vi "Auto Resize All Tree Columns (Uniform Text).vi"(6 "IngoreCols(Empty as default)":i32[](array[numeric]), 8 "error in (no error)":errorcluster, 11 "Tree Control":refnum<vi>) -> (0 "error out":errorcluster, 3 "Tree Control":refnum<vi>)   [LabVIEW 2017, in "csm-ui-support.lvlib"]
doc: "This VI resizes each column of the Tree specified by Tree Ref based on the widest entry of the column. Additionally, the array based on the Tree can be calculated according to the Tree Ref, which don't need additional input."
uses:
  csm-ui-support.lvlib
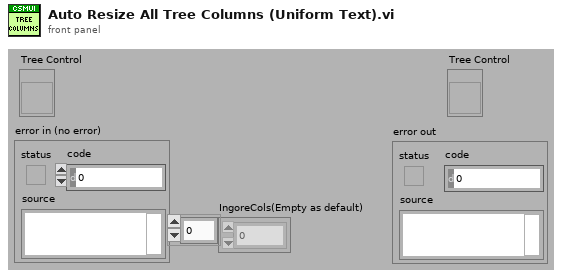
[diagram p1: front panel]
types:
  T1 = cluster{"Font Name:":string, "Size":i16, "Strikeout?":bool, "Italic?":bool, "Underline?":bool, "Outline?":bool, "Shadow?":bool, "Bold?":bool}
  T2 = enum16{"User-specified Font", "Application Font", "System Font", "Dialog Font"}
  T3 = cluster{"left":i16, "top":i16, "right":i16, "bottom":i16}
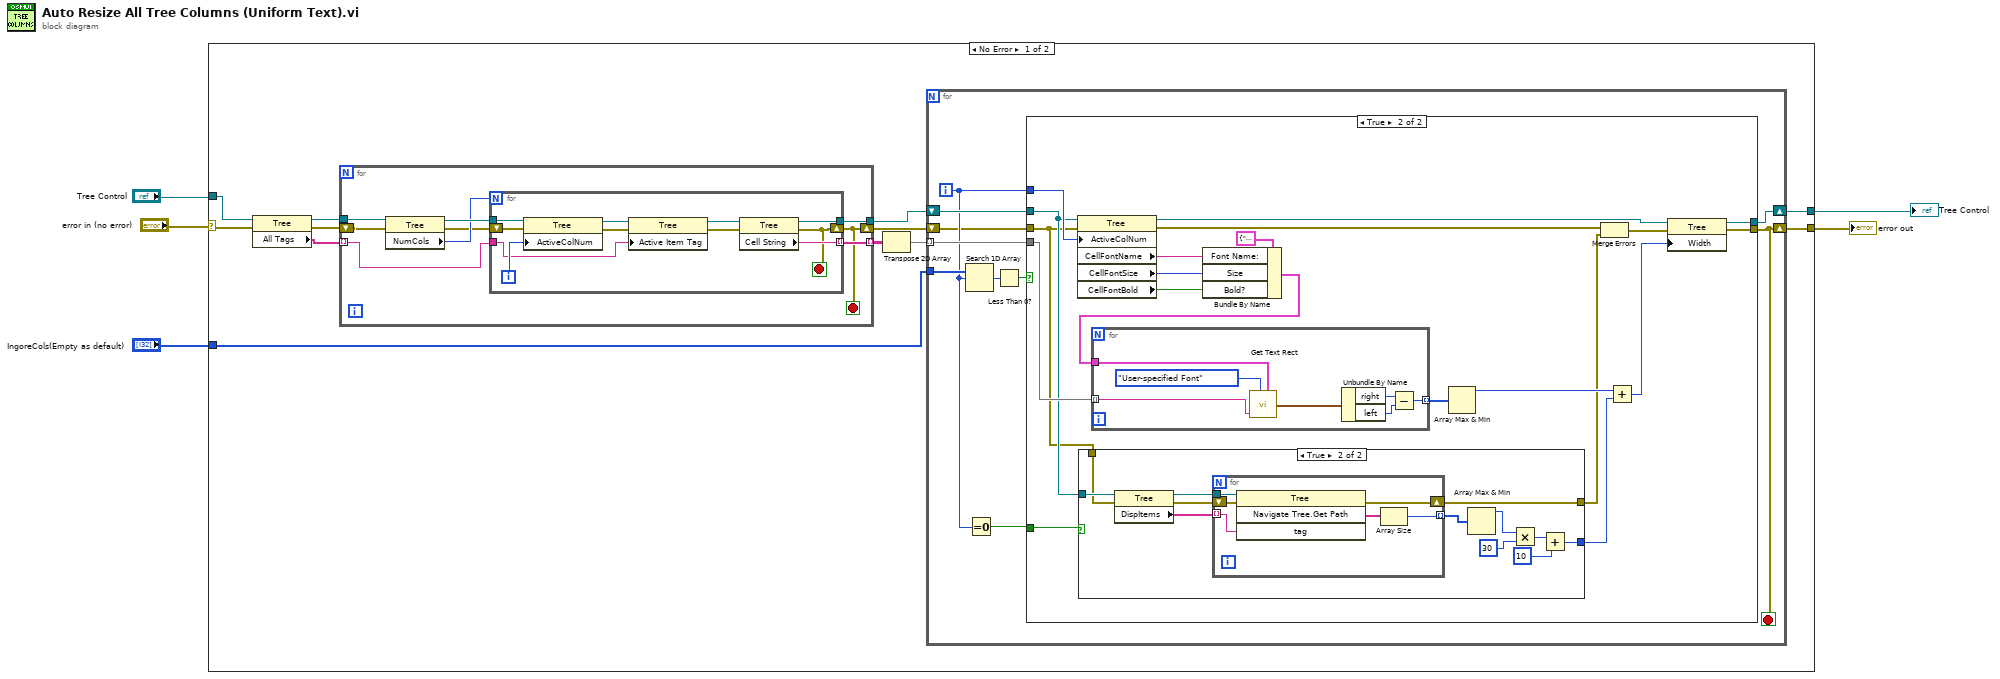
[diagram p0: block diagram]
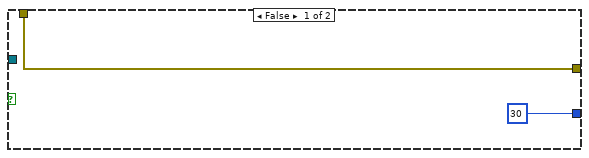
[diagram p3: hidden frame]
diagram:
  n1 = case shown="No Error" "error in (no error)" {
    selector: "error in (no error)" -> [w9 w97]
    tunnel: "Tree Control" -> [w12 w98]
    tunnel: [w11 w98] -> w2
    tunnel: [w6 w97] -> w1
    tunnel: "IngoreCols(Empty as default)" -> [w10 _]
    frame No Error {
      n2 = property class="Tree"(reference=w12, error in=w9) -> (reference out=w16:refnum<vi>, error out=w8:errorcluster, "All Tags"=w17:string[])
      n3 = for {
        tunnel: w17 -> [w22] mode=indexing
        tunnel: [w26] -> w15 mode=indexing
        tunnel: w16 -> [w25]
        tunnel: [w24] -> w14
        shift-right: [w18] -> w7
        shift-left: w8 -> [w20]
        stop <- w18 stop-if-true
        n4 = property class="Tree"(reference=w25, error in=w20) -> (reference out=w23:refnum<vi>, error out=w19:errorcluster, "NumCols"=w21:u32)
        n5 = for {
          N: w21 -> [_]
          tunnel: w22 -> [w31]
          tunnel: [w37] -> w26 mode=indexing
          tunnel: w23 -> [w36]
          tunnel: [w35] -> w24
          shift-right: [w27] -> w18
          shift-left: w19 -> [w28]
          i -> [w33]
          stop <- w27 stop-if-true
          n6 = property class="Tree"(reference=w36, error in=w28, "ActiveColNum"=w33) -> (reference out=w34:refnum<vi>, error out=w30:errorcluster)
          n7 = property class="Tree"(reference=w34, error in=w30, "Active Item Tag"=w31) -> (reference out=w32:refnum<vi>, error out=w29:errorcluster)
          n8 = property class="Tree"(reference=w32, error in=w29) -> (reference out=w35:refnum<vi>, error out=w27:errorcluster, "Cell String"=w37:string)
        }
      }
      n9 = Transpose 2D Array(2D array=w15) -> (transposed array=w13:string[][])
      n10 = for {
        tunnel: w13 -> [w47] mode=indexing
        shift-right: [w46] -> w11
        shift-left: w14 -> [w44]
        tunnel: w10 -> [w41]
        shift-right: [w38] -> w6
        shift-left: w7 -> [w39]
        i -> [w40]
        stop <- w38 stop-if-true
        n11 = Search 1D Array(1D array=w41, element=w40) -> (index of element=w43:i32)  [unwired: 1 in]
        n12 = Equal To 0?(x=w40) -> (x = 0?=w45:bool)
        n13 = Less Than 0?(x=w43) -> (x < 0?=w42:bool)
        n14 = case shown="True" w42 {
          tunnel: w47 -> [_ w69]
          tunnel: [w49 w68] -> w46
          tunnel: w40 -> [_ w59]
          tunnel: w45 -> [_ w58]
          tunnel: w44 -> [w49 w56]
          tunnel: w39 -> [w48 w54]
          tunnel: [w48 w50] -> w38
          frame False {
          }
          frame True {
            n15 = property class="Tree"(reference=w56, error in=w54, "ActiveColNum"=w59) -> (reference out=w60:refnum<vi>, error out=w51:errorcluster, "CellFontName"=w65:string, "CellFontSize"=w63:u32, "CellFontBold"=w64:bool)
            n16 = case shown="True" w58 {
              tunnel: [30 w80] -> w57
              tunnel: w56 -> [_ w79]
              tunnel: w54 -> [w70 w74]
              tunnel: [w70 w72] -> w52
              frame False {
              }
              frame True {
                n17 = property class="Tree"(reference=w79, error in=w74) -> (reference out=w77:refnum<vi>, error out=w73:errorcluster, "DispItems"=w78:string[])
                n18 = for {
                  tunnel: w78 -> [w88] mode=indexing
                  tunnel: w77 -> [w89]
                  tunnel: [w86] -> w76 mode=indexing
                  shift-right: [w84] -> w72
                  shift-left: w73 -> [w85]
                  n19 = invoke class="Tree" method="Navigate Tree.Get Path"(reference=w89, error in=w85, "tag"=w88) -> (error out=w84:errorcluster, "Navigate Tree:Get Path"=w87:string[])  [unwired: 1 in, 2 out]
                  n20 = Array Size(array=w87) -> (size(s)=w86:i32)
                }
                n21 = Array Max & Min(array=w76) -> (max value=w75:i32)  [unwired: 3 out]
                n22 = Multiply(x=w75, y=30) -> (x*y=w82:i32)
                n23 = Add(x=w82, y=10) -> (x+y=w80:i32)
              }
            }
            n24 = Bundle By Name(cluster=T1 {"Font Name:"="", "Size"=0, "Strikeout?"=FALSE, "Italic?"=FALSE, "Underline?"=FALSE, "Outline?"=FALSE, "Shadow?"=FALSE, "Bold?"=FALSE} ("[user-specified font]"), "Font Name:"=w65, "Size"=w63, "Bold?"=w64) -> (w61:T1)
            n25 = for {
              tunnel: w69 -> [w96] mode=indexing
              tunnel: [w92] -> w67 mode=indexing
              tunnel: w61 -> [w91]
              n26 = call <vilib>:"Get Text Rect.vi"("desired font(Application)"=T2."User-specified Font", "text"=w96, "[user-specified font]"=w91) -> ("rect"=w95:T3)  [unwired: 6 in]
              n27 = Unbundle By Name(w95) -> ("right"=w94:i16, "left"=w93:i16)
              n28 = Subtract(x=w94, y=w93) -> (x-y=w92:i16)
            }
            n29 = Array Max & Min(array=w67) -> (max value=w66:i16)  [unwired: 3 out]
            n30 = Merge Errors(w51, w52) -> (w53:errorcluster)
            n31 = Add(x=w66, y=w57) -> (x+y=w55:i32)
            n32 = property on="Property Node" class="Tree"(reference=w60, error in=w53, "Width"=w55) -> (reference out=w68:refnum<vi>, error out=w50:errorcluster)
          }
        }
      }
    }
    frame Error {
    }
  }
  "error out" <- w1
  "Tree Control" <- w2
